vi "Express VI - Statistics.vi"() -> ()   [LabVIEW 2023]
doc: "This example shows the results of statistical functions. There is a Histogram of all values and there is the Minimum, Maximum and Mean for each packet of data.\n\nThis example uses the following Express VIs: Simulate Signal, Create Histogram, and Statistics."
uses:
  Instance           1 18Saved   Statistics .vi
  Instance           3 18Saved   Statistics .vi
  Instance           2 18Saved   Statistics .vi
panel:
  out "Chart":dynamicdata(graph)
  out "Mean":dbl
  out "Minimum":dbl
  out "Maximum":dbl
  out "Signal":dynamicdata(graph)
  out "Histogram":dynamicdata(graph)
  in  "Stop":bool
  # "Overview: Shows the results of the Statistics Express VI.\nRequirements: LabVIEW Full Development System\nInstructions:\n1. Run the VI.\n2. View the simulated signal (Gaussian noise).\n3. There is a histogram of all values. The chart displays the minimum, maximum and mean for each packet of data.\n4. Click Stop to stop the VI."
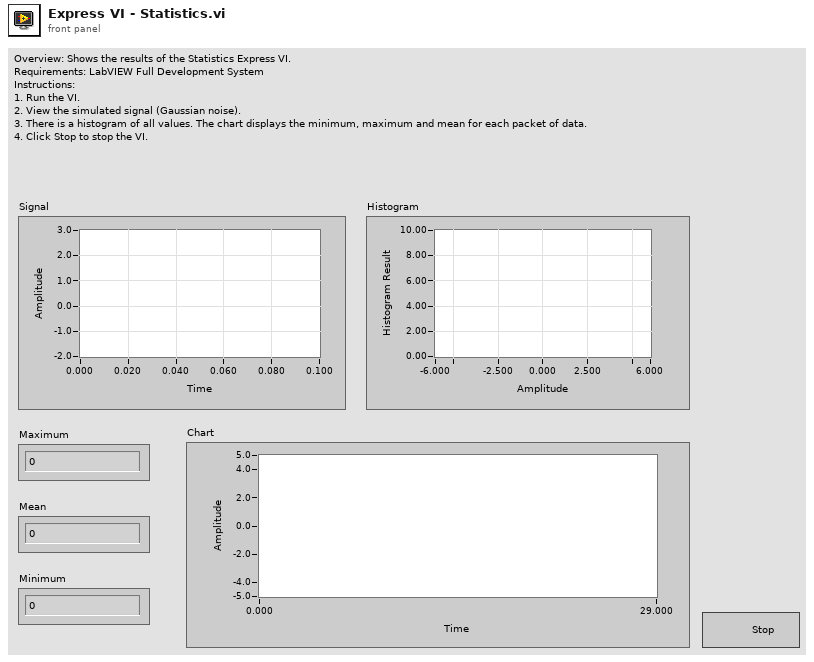
[diagram p1: front panel]
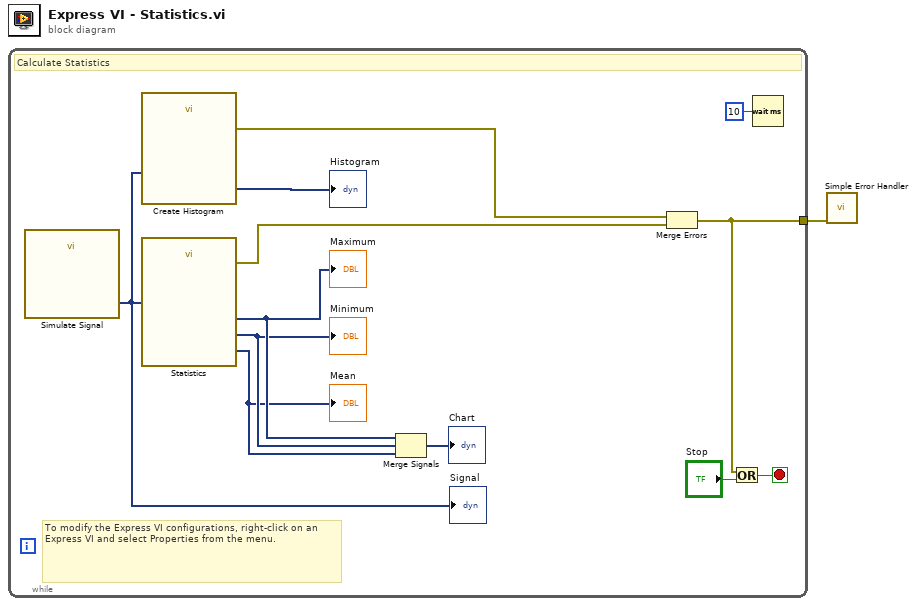
[diagram p0: block diagram]
diagram:
  n1 = while {
    tunnel: [w2] -> w1
    stop <- w3 stop-if-true
    # "To modify the Express VI configurations, right-click on an Express VI and select Properties from the menu."
    # "Calculate Statistics"
    n2 = call "Simulate Signal"() -> ("DC with Gaussian Noise"=w10:dynamicdata)  [unwired: 14 in, 1 out]
    "Signal" <- w10
    n3 = call "Create Histogram"("Signal"=w10) -> ("error out"=w5:errorcluster, "Histogram"=→"Histogram":dynamicdata)  [unwired: 9 in]
    n4 = call "Statistics"("Signals"=w10) -> ("Arithmetic Mean"=w7:dynamicdata, "Minimum"=w8:dynamicdata, "Maximum"=w9:dynamicdata, "error out"=w4:errorcluster)  [unwired: 23 in]
    "Maximum" <- w9
    "Minimum" <- w8
    "Mean" <- w7
    n5 = Merge Signals(w9, w8, w7) -> (→"Chart":dynamicdata)
    n6 = Merge Errors(w5, w4) -> (w2:errorcluster)
    n7 = Or(x=w2, y="Stop") -> (x .or. y?=w3:bool)
    n8 = Wait (ms)(milliseconds to wait=u32 10) -> ()  [unwired: 1 out]
  }
  n9 = call <vilib>:"Simple Error Handler.vi"("error in (no error)"=w1) -> ()  [unwired: 4 in, 5 out]
